vi "InitialFileFolderCreation_V2.vi"(6 "New Run?":bool, 8 "error in (no error)":errorcluster, 9 "Run Number":string, 10 "Subfolders&NumChannelsRecorded":cluster{"subfolder":string, i32}[](array[cluster]), 11 "base path":path) -> (0 "error out":errorcluster, 1 "SupplementalDataFileReferenceObjectArrayWsubfolders":refnum<file>[][](array[refnum]), 2 "DataFileReferenceObjectArrayWsubfolders":refnum<file>[][](array[refnum]), 3 "created path array":path[](array[path]))   [LabVIEW 2019]
panel:
  out "DataFileReferenceObjectArray":refnum<file>[](array[refnum])
  out "created path":path
  out "SupplementalDataFileReferenceObjectArray":refnum<file>[](array[refnum])
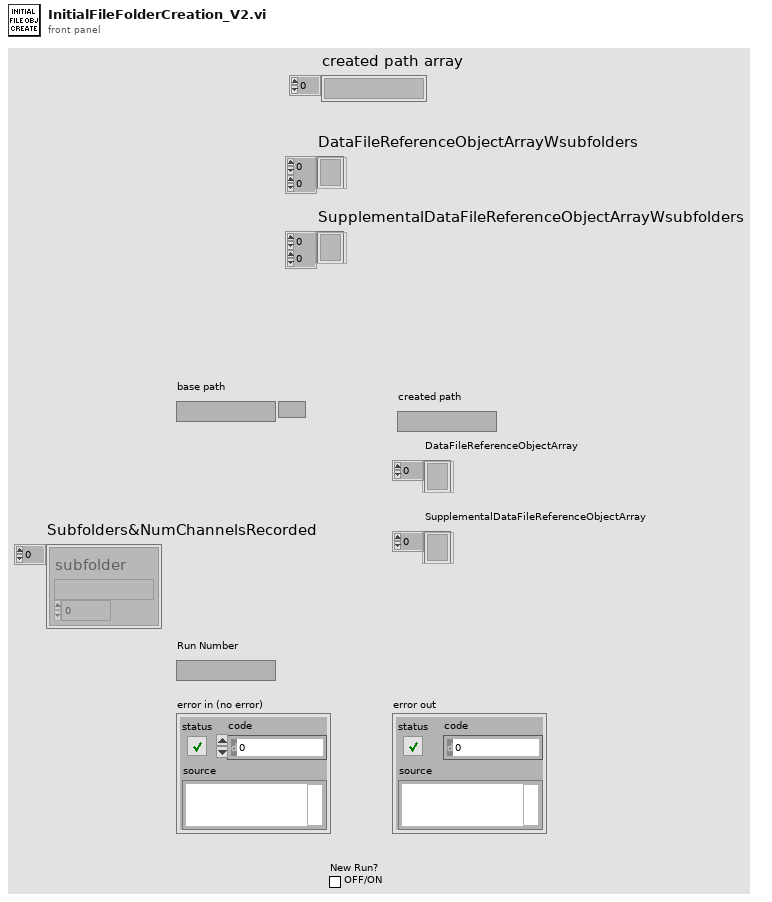
[diagram p1: front panel]
types:
  T1 = enum16{"open", "replace", "create", "open or create", "replace or create", "replace or create with confirmation"}
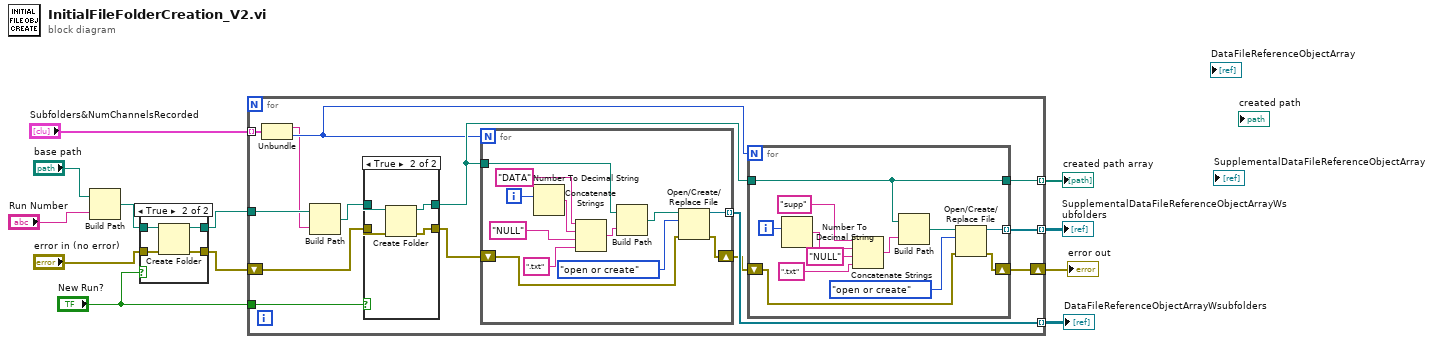
[diagram p0: block diagram]
diagram:
  n1 = Build Path(base path="base path", name or relative path="Run Number") -> (appended path=w5:path)
  n2 = case shown="True" "New Run?" {
    tunnel: "error in (no error)" -> [w13 w18]
    tunnel: [w13 w15] -> w3
    tunnel: [w14 w16] -> w4
    tunnel: w5 -> [w14 w17]
    frame False {
    }
    frame True {
      n3 = Create Folder(path (use dialog)=w17, error in=w18) -> (created path=w16:path, error out=w15:errorcluster)  [unwired: 1 in, 1 out]
    }
  }
  n4 = for {
    tunnel: [w32] -> w7 mode=indexing
    tunnel: [w30] -> w6 mode=indexing
    tunnel: "New Run?" -> [w27]
    shift-right: [w29] -> w11
    shift-left: w3 -> [w21]
    tunnel: "Subfolders&NumChannelsRecorded" -> [w24] mode=indexing
    tunnel: w4 -> [w22]
    tunnel: [w31] -> w12 mode=indexing
    n5 = Unbundle(w24) -> ("subfolder"=w20:string, w23:i32)
    n6 = Build Path(base path=w22, name or relative path=w20) -> (appended path=w19:path)
    n7 = case shown="True" w27 {
      tunnel: w21 -> [w33 w35]
      tunnel: [w33 w37] -> w26
      tunnel: [w34 w38] -> w25
      tunnel: w19 -> [w34 w36]
      frame False {
      }
      frame True {
        n8 = Create Folder(path (use dialog)=w36, error in=w35) -> (created path=w38:path, error out=w37:errorcluster)  [unwired: 1 in, 1 out]
      }
    }
    n9 = for {
      N: w23 -> [_]
      tunnel: w25 -> [w58]
      shift-right: [w56] -> w28
      shift-left: w26 -> [w57]
      tunnel: [w55] -> w30 mode=indexing
      i -> [w54]
      n10 = Number To Decimal String(number=w54) -> (decimal integer string=w51:string)  [unwired: 1 in]
      n11 = Concatenate Strings("DATA" ("string"), w51, "NULL" ("string"), ".txt" ("string")) -> (w62:string)
      n12 = Build Path(base path=w58, name or relative path=w62) -> (appended path=w61:path)
      n13 = Open/Create/Replace File(file path (use dialog)=w61, error in=w57, operation (0:open)=T1."open or create") -> (refnum out=w55:refnum<file>, error out=w56:errorcluster)  [unwired: 3 in, 1 out]
    }
    n14 = for {
      N: w23 -> [_]
      tunnel: w25 -> [w43]
      shift-right: [w45] -> w29
      shift-left: w28 -> [w46]
      tunnel: [w44] -> w32 mode=indexing
      tunnel: [w43] -> w31
      i -> [w42]
      n15 = Number To Decimal String(number=w42) -> (decimal integer string=w40:string)  [unwired: 1 in]
      n16 = Concatenate Strings("supp" ("string"), w40, "NULL" ("string"), ".txt" ("string")) -> (w50:string)
      n17 = Build Path(base path=w43, name or relative path=w50) -> (appended path=w49:path)
      n18 = Open/Create/Replace File(file path (use dialog)=w49, error in=w46, operation (0:open)=T1."open or create") -> (refnum out=w44:refnum<file>, error out=w45:errorcluster)  [unwired: 3 in, 1 out]
    }
  }
  "error out" <- w11
  "SupplementalDataFileReferenceObjectArrayWsubfolders" <- w7
  "DataFileReferenceObjectArrayWsubfolders" <- w6
  "created path array" <- w12
